vi "Opt3.vi"(0 "Activation Function":enum32{"Sigmoid", "RELU", "Tanh", "Leaky RELU"}(ring), 1 "Weights l+1":dbl[][](array[numeric]), 2 "Weights":dbl[][](array[numeric]), 3 "Biases":dbl[](array[numeric]), 5 "Net Output":dbl[](array[numeric]), 7 "Activations l-1":dbl[](array[numeric]) format="%.2f", 9 "Delta l+1":dbl[](array[numeric])) -> (13 "Updated Weights":dbl[][](array[numeric]), 14 "Updated Biases":dbl[](array[numeric]))   [LabVIEW 2018]
uses:
  <vilib>/Analysis/baseanly.llb/A x Vector.vi
  <vilib>/Analysis/baseanly.llb/Real Outer Product.vi
  <vilib>/Analysis/Matrix/Numeric/Conversions/Matrix To Array - RM.vi
  Optimizer.vi
  Adam_data.vi
  Iteration Counter.vi
  <vilib>/Analysis/NI_AALBase.lvlib
  <vilib>/Analysis/Matrix/NI_Matrix.lvlib
panel:
  out "Grad. w":dbl[][](array[numeric])
  out "Grad. b":dbl[](array[numeric])
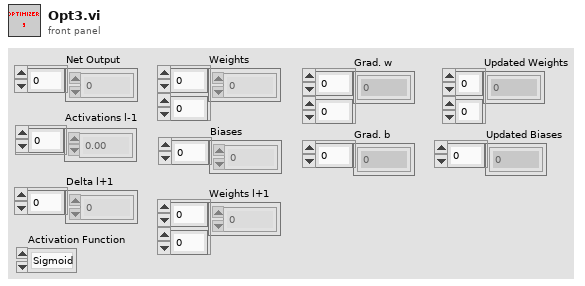
[diagram p1: front panel]
types:
  T1 = typedef "NI_Matrix.lvlib/RealMatrix.ctl" = dbl[][]
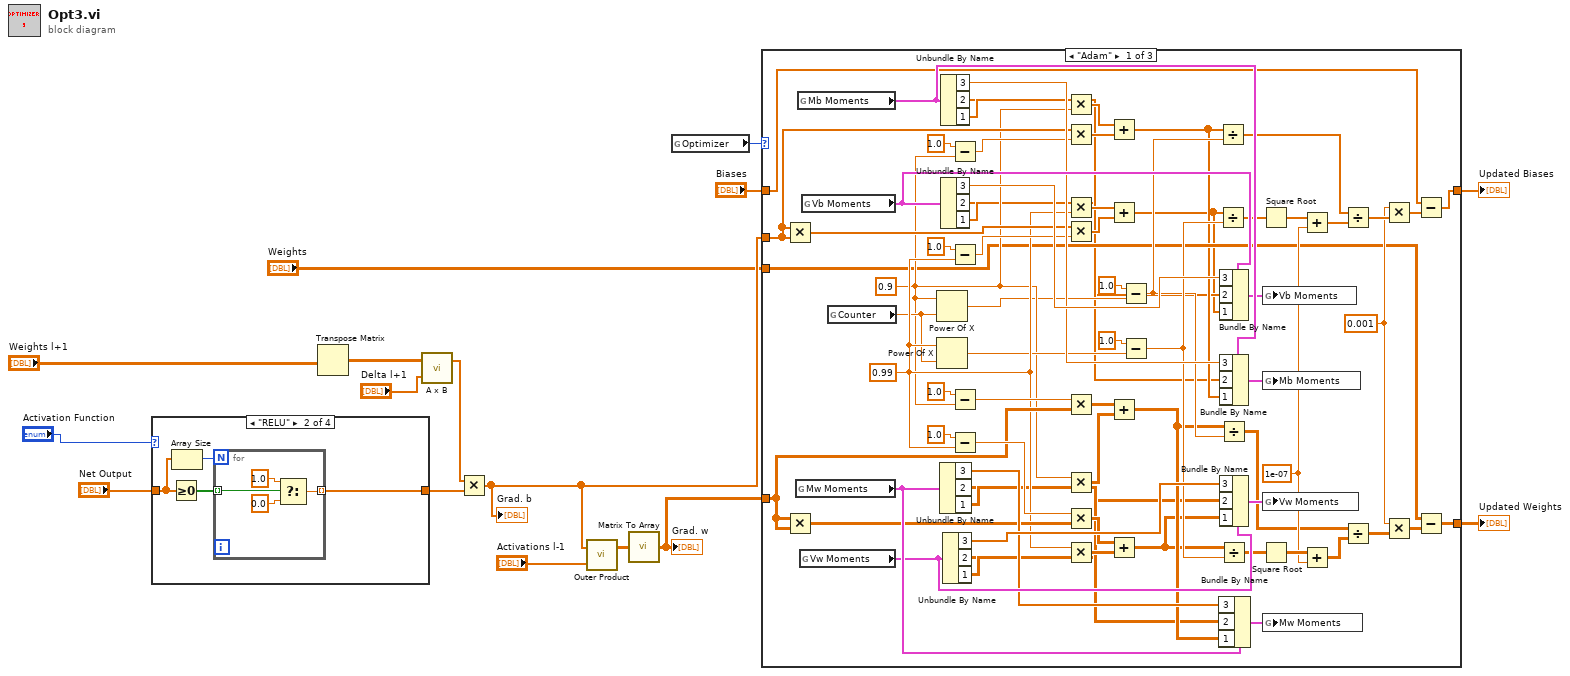
[diagram p0: block diagram]
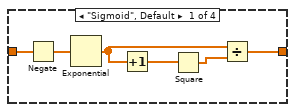
[diagram p4: hidden frame]
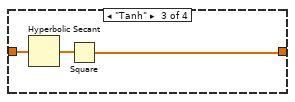
[diagram p5: hidden frame]
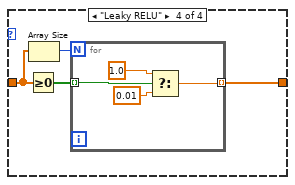
[diagram p6: hidden frame]
diagram:
  n1 = case shown="\"RELU\"" "Activation Function" {
    tunnel: "Net Output" -> [w18 w24 w32 w35]
    tunnel: [w17 w26 w31 w37] -> w15
    frame "Sigmoid", Default {
      n2 = Negate(x=w18) -> (-x=w22:dbl[])
      n3 = Exponential(1:w22) -> (0:w19:dbl[])
      n4 = Increment(x=w19) -> (x+1=w21:dbl[])
      n5 = Square(x=w21) -> (x^2=w20:dbl[])
      n6 = Divide(x=w19, y=w20) -> (x/y=w17:dbl[])
    }
    frame "RELU" {
      n7 = Greater Or Equal To 0?(x=w24) -> (x >= 0?=w25:bool[])
      n8 = Array Size(array=w24) -> (size(s)=w23:i32)
      n9 = for {
        N: w23 -> [_]
        tunnel: [w30] -> w26 mode=indexing
        tunnel: w25 -> [w27] mode=indexing
        n10 = Select(t=1.0, s=w27, f=0.0) -> (s? t:f=w30:dbl)
      }
    }
    frame "Tanh" {
      n11 = Hyperbolic Secant(1:w32) -> (0:w33:dbl[])
      n12 = Square(x=w33) -> (x^2=w31:dbl[])
    }
    frame "Leaky RELU" {
      n13 = Greater Or Equal To 0?(x=w35) -> (x >= 0?=w36:bool[])
      n14 = Array Size(array=w35) -> (size(s)=w34:i32)
      n15 = for {
        N: w34 -> [_]
        tunnel: [w39] -> w37 mode=indexing
        tunnel: w36 -> [w38] mode=indexing
        n16 = Select(t=1.0, s=w38, f=0.01) -> (s? t:f=w39:dbl)
      }
    }
  }
  n17 = Transpose Matrix(1:"Weights l+1") -> (0:w11:dbl[][])
  n18 = call-poly <vilib>:"A x B.vi"("Vector"="Delta l+1", "A"=w11) -> ("A x Vector"=w9:dbl[])  [unwired: 1 out]
  n19 = Multiply(x=w9, y=w15) -> (x*y=w7:dbl[])
  "Grad. b" <- w7
  n20 = call-poly <vilib>:"Outer Product.vi"("Y Vector"="Activations l-1", "X Vector"=w7) -> ("Outer Product"=w6:T1)  [unwired: 1 out]
  n21 = call-poly <vilib>:"Matrix To Array.vi"("Real Matrix"=w6) -> ("Real 2D Array"=w5:dbl[][])
  "Grad. w" <- w5
  n22 = global read "Optimizer.vi" "Optimizer"() -> (w14:enum16{"Adagrad", "Adadelta", "Adam"})
  n23 = case shown="\"Adam\"" w14 {
    tunnel: "Weights" -> [w55 w114 w116]
    tunnel: [w54 w114 w116] -> w4
    tunnel: "Biases" -> [w58 w113 w115]
    tunnel: [w57 w113 w115] -> w12
    tunnel: w7 -> [w96 _ _]
    tunnel: w5 -> [w83 _ _]
    frame "Adam" {
      w64 = 1e-07
      w60 = 0.001
      w80 = 0.99
      w76 = 0.9
      n24 = Multiply(x=w96, y=w96) -> (x*y=w95:dbl[])
      n25 = Multiply(x=w83, y=w83) -> (x*y=w86:dbl[][])
      n26 = global read "Adam_data.vi" "Mw Moments"() -> (w111:cluster{"3 ":dbl[], "2":dbl[][], "1":dbl[][]})
      n27 = global read "Adam_data.vi" "Mb Moments"() -> (w108:cluster{"1":dbl[], "2":dbl[], "3":dbl})
      n28 = global read "Adam_data.vi" "Vw Moments"() -> (w110:cluster{"3":dbl[], "2":dbl[][], "1":dbl[][]})
      n29 = global read "Adam_data.vi" "Vb Moments"() -> (w106:cluster{"3":dbl, "2":dbl[], "1":dbl[]})
      n30 = global read "Iteration Counter.vi" "Counter"() -> (w77:dbl)
      n31 = Power Of X(1:w77, 2:w76) -> (0:w74:dbl)
      n32 = Power Of X(1:w77, 2:w80) -> (0:w79:dbl)
      n33 = Unbundle By Name(w111) -> ("3"=w91:dbl[], "2"=w45:dbl[][], "1"=w47:dbl[][])
      n34 = Unbundle By Name(w108) -> ("3"=w103:dbl, "2"=w51:dbl[], "1"=w53:dbl[])
      n35 = Unbundle By Name(w106) -> ("3"=w104:dbl, "2"=w49:dbl[], "1"=w50:dbl[])
      n36 = Unbundle By Name(w110) -> ("3"=w92:dbl[], "2"=w42:dbl[][], "1"=w44:dbl[][])
      n37 = Subtract(x=1.0, y=w76) -> (x-y=w101:dbl)
      n38 = Subtract(x=1.0, y=w80) -> (x-y=w97:dbl)
      n39 = Subtract(x=1.0, y=w76) -> (x-y=w84:dbl)
      n40 = Subtract(x=1.0, y=w80) -> (x-y=w89:dbl)
      n41 = Multiply(x=w53, y=w76) -> (x*y=w100:dbl[])
      n42 = Multiply(x=w96, y=w101) -> (x*y=w99:dbl[])
      n43 = Multiply(x=w50, y=w80) -> (x*y=w94:dbl[])
      n44 = Multiply(x=w95, y=w97) -> (x*y=w93:dbl[])
      n45 = Multiply(x=w84, y=w83) -> (x*y=w82:dbl[][])
      n46 = Multiply(x=w76, y=w47) -> (x*y=w81:dbl[][])
      n47 = Multiply ("Multiply.vi")(x=w89, y=w86) -> (x*y=w88:dbl[][])
      n48 = Multiply(x=w80, y=w44) -> (x*y=w87:dbl[][])
      n49 = Add(x=w100, y=w99) -> (x+y=w52:dbl[])
      n50 = Add(x=w94, y=w93) -> (x+y=w48:dbl[])
      n51 = Add(x=w82, y=w81) -> (x+y=w46:dbl[][])
      n52 = Add(x=w88, y=w87) -> (x+y=w43:dbl[][])
      n53 = Subtract(x=1.0, y=w74) -> (x-y=w72:dbl)
      n54 = Subtract(x=1.0, y=w79) -> (x-y=w73:dbl)
      n55 = Divide(x=w52, y=w72) -> (x/y=w68:dbl[])
      n56 = Divide(x=w48, y=w73) -> (x/y=w71:dbl[])
      n57 = Divide(x=w46, y=w72) -> (x/y=w63:dbl[][])
      n58 = Divide(x=w43, y=w73) -> (x/y=w66:dbl[][])
      n59 = Bundle By Name(cluster=w111, "3"=w91, "2"=w45, "1"=w46) -> (w112:cluster{"3 ":dbl[], "2":dbl[][], "1":dbl[][]})
      n60 = Bundle By Name(cluster=w106, "3"=w104, "2"=w49, "1"=w48) -> (w105:cluster{"3":dbl, "2":dbl[], "1":dbl[]})
      n61 = Bundle By Name(cluster=w108, "3"=w103, "2"=w51, "1"=w52) -> (w107:cluster{"1":dbl[], "2":dbl[], "3":dbl})
      n62 = Bundle By Name(cluster=w110, "3"=w92, "2"=w42, "1"=w43) -> (w109:cluster{"3":dbl[], "2":dbl[][], "1":dbl[][]})
      n63 = Square Root(x=w71) -> (sqrt(x)=w70:dbl[])
      n64 = Square Root(x=w66) -> (sqrt(x)=w65:dbl[][])
      n65 = global write "Adam_data.vi" "Vb Moments"(w105) -> ()
      n66 = global write "Adam_data.vi" "Mb Moments"(w107) -> ()
      n67 = global write "Adam_data.vi" "Vw Moments"(w109) -> ()
      n68 = global write "Adam_data.vi" "Mw Moments"(w112) -> ()
      n69 = Add(x=w70, y=w64) -> (x+y=w69:dbl[])
      n70 = Add(x=w65, y=w64) -> (x+y=w62:dbl[][])
      n71 = Divide(x=w68, y=w69) -> (x/y=w67:dbl[])
      n72 = Divide(x=w63, y=w62) -> (x/y=w61:dbl[][])
      n73 = Multiply(x=w60, y=w67) -> (x*y=w59:dbl[])
      n74 = Multiply(x=w60, y=w61) -> (x*y=w56:dbl[][])
      n75 = Subtract(x=w58, y=w59) -> (x-y=w57:dbl[])
      n76 = Subtract(x=w55, y=w56) -> (x-y=w54:dbl[][])
    }
    frame "Adadelta" {
    }
    frame "Adagrad" {
    }
  }
  "Updated Biases" <- w12
  "Updated Weights" <- w4
